vi "KE6221 -- Get Wave Offset.vi"(0 "Resource In":refnum<visa-resource-name>, 1 "Check For SCPI Errors? (T)":bool=TRUE, 11 "error in (no error)":errorcluster) -> (4 "Resource Out (dupl)":refnum<visa-resource-name>, 8 "Wave Offset (A)":T1=0.1 min=-0.105 max=0.105 format="%.4p", 15 "error out":errorcluster)   [LabVIEW 2020, in "Keithley 622x.lvlib"]
uses:
  Keithley 622x.lvlib
  Source/Typedefs/KE622x -- Current Level.ctl
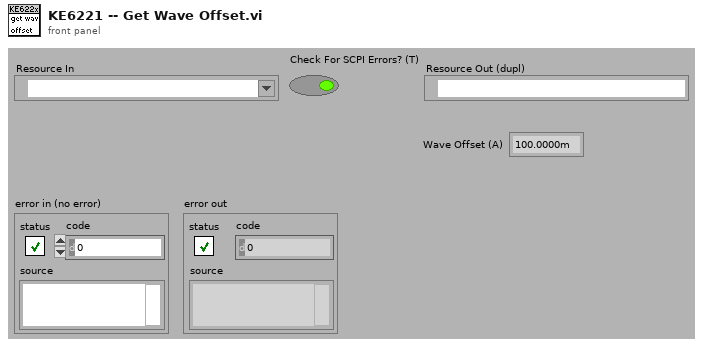
[diagram p1: front panel]
types:
  T1 = typedef "Keithley 622x.lvlib/KE622x -- Current Level.ctl" = dbl
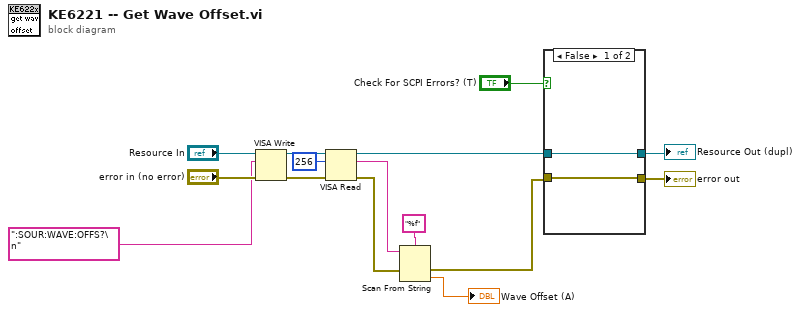
[diagram p0: block diagram]
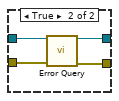
[diagram p2: hidden frame]
diagram:
  n1 = VISA Write(VISA resource name="Resource In", write buffer=":SOUR:WAVE:OFFS?\n" ("format string"), error in (no error)="error in (no error)") -> (VISA resource name out=w9:refnum<visa-resource-name>, error out=w8:errorcluster)  [unwired: 1 out]
  n2 = VISA Read(VISA resource name=w9, byte count=u32 256, error in (no error)=w8) -> (VISA resource name out=w2:refnum<visa-resource-name>, read buffer=w4:string, error out=w6:errorcluster)  [unwired: 1 out]
  n3 = Scan From String(format string="%f", input string=w4, error in=w6) -> (error out=w3:errorcluster, output 1=→"Wave Offset (A)":T1)  [unwired: 2 in, 2 out]
  n4 = case shown="False" "Check For SCPI Errors? (T)" {
    tunnel: w2 -> [w17 w21]
    tunnel: w3 -> [w16 w20]
    tunnel: [w16 w19] -> w11
    tunnel: [w17 w18] -> w12
    frame False {
    }
    frame True {
      n5 = call "Error Query.vi"("VISA Resource In"=w21, "error in (no error)"=w20) -> ("VISA Resource Out (dupl)"=w18:refnum<visa-resource-name>, "error out"=w19:errorcluster)  [unwired: 10 in, 2 out]
    }
  }
  "Resource Out (dupl)" <- w12
  "error out" <- w11
